vi "Multiclamp Capacitance Compensation.vi"(7 "#i":i32, 8 "error in (no error)":errorcluster, 9 "Timeout [ms]":u32, 10 "pnError":i32, 11 "hMCCmsg":i32) -> (0 "error out":errorcluster, 2 "pnError out":i32, 3 "Handler":i32)   [LabVIEW 2012, in "MultiClamp 700B Controls.lvlib"]
uses:
  MultiClamp 700B Controls.lvlib
  AxMultiClampMsg/AxMultiClampMsg.lvlib
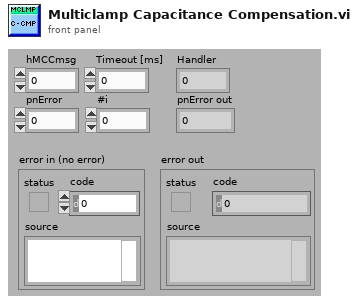
[diagram p1: front panel]
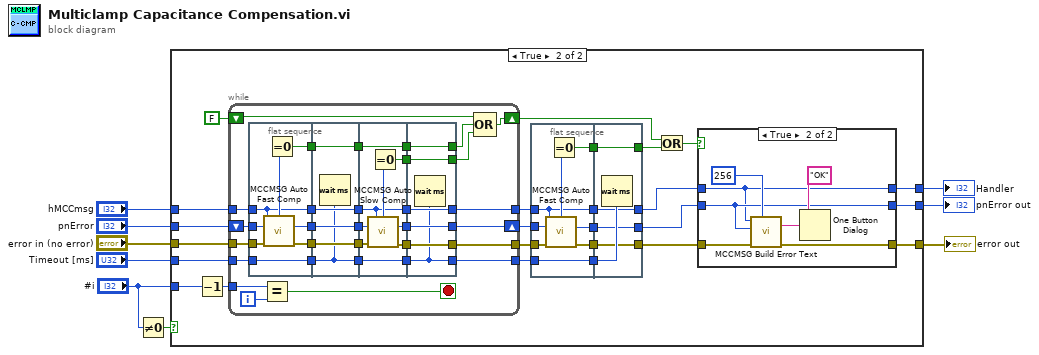
[diagram p0: block diagram]
diagram:
  n1 = Not Equal To 0?(x="#i") -> (x != 0?=w2:bool)
  n2 = case shown="True" w2 {
    tunnel: [w12 w32] -> w9
    tunnel: [w11 w31] -> w8
    tunnel: [w10 w30] -> w7
    tunnel: "error in (no error)" -> [w12 w29]
    tunnel: "pnError" -> [w10 w28]
    tunnel: "Timeout [ms]" -> [_ w27]
    tunnel: "#i" -> [_ w15]
    tunnel: "hMCCmsg" -> [w11 w13]
    frame False {
    }
    frame True {
      n3 = Decrement(x=w15) -> (x-1=w14:i32)
      n4 = while {
        tunnel: [w54] -> w25
        tunnel: [w52] -> w19
        tunnel: w29 -> [w63]
        tunnel: w13 -> [w62]
        tunnel: w27 -> [w60]
        tunnel: w14 -> [w59]
        shift-right: [w53] -> w23
        shift-left: w28 -> [w61]
        shift-right: [w56] -> w18
        shift-left: FALSE -> [w55]
        tunnel: [w51] -> w24
        i -> [w58]
        stop <- w57 stop-if-true
        n5 = flat-sequence {
          tunnel: [w89] -> w81
          tunnel: [w88] -> w80
          tunnel: w62 -> [w83]
          tunnel: w61 -> [w87]
          tunnel: w63 -> [w86]
          tunnel: [w84] -> w79
          tunnel: [w83] -> w78
          tunnel: w60 -> [w82]
          tunnel: [w82] -> w77
          tunnel: [w94] -> w76
          tunnel: w81 -> [w94]
          tunnel: w80 -> [w93]
          tunnel: [w93] -> w75
          tunnel: [w92] -> w74
          tunnel: w79 -> [w92]
          tunnel: [w91] -> w73
          tunnel: w78 -> [w91]
          tunnel: w77 -> [w90]
          tunnel: [w90] -> w72
          tunnel: w76 -> [w103]
          tunnel: [w102] -> w71
          tunnel: [w101] -> w70
          tunnel: w75 -> [w100]
          tunnel: [w98] -> w69
          tunnel: w74 -> [w98]
          tunnel: [w97] -> w68
          tunnel: w73 -> [w96]
          tunnel: [w96] -> w67
          tunnel: w72 -> [w95]
          tunnel: [w95] -> w66
          tunnel: w71 -> [w107]
          tunnel: w70 -> [w106]
          tunnel: w69 -> [w109]
          tunnel: w68 -> [w108]
          tunnel: w67 -> [w105]
          tunnel: w66 -> [w104]
          tunnel: [w109] -> w65
          tunnel: [w108] -> w64
          tunnel: [w107] -> w54
          tunnel: [w106] -> w53
          tunnel: [w105] -> w52
          tunnel: [w104] -> w51
          frame #0 {
            n6 = call "MCCMSG Auto Fast Comp.vi"("error in (no error)"=w86, "pnError"=w87, "hMCCmsg"=w83) -> ("error out"=w89:errorcluster, "pnError out"=w88:i32, "function return"=w85:i32)  [unwired: 6 in]
            n7 = Equal To 0?(x=w85) -> (x = 0?=w84:bool)
          }
          frame #1 {
            n8 = Wait (ms)(milliseconds to wait=w90) -> ()  [unwired: 1 out]
          }
          frame #2 {
            n9 = call "MCCMSG Auto Slow Comp.vi"("error in (no error)"=w103, "pnError"=w100, "hMCCmsg"=w96) -> ("error out"=w102:errorcluster, "pnError out"=w101:i32, "function return"=w99:i32)  [unwired: 6 in]
            n10 = Equal To 0?(x=w99) -> (x = 0?=w97:bool)
          }
          frame #3 {
            n11 = Wait (ms)(milliseconds to wait=w104) -> ()  [unwired: 1 out]
          }
        }
        n12 = Equal?(x=w59, y=w58) -> (x = y?=w57:bool)
        n13 = Compound Arithmetic op=OR(w55, w65, w64) -> (w56:bool)
      }
      n14 = flat-sequence {
        tunnel: [w45] -> w37
        tunnel: [w44] -> w36
        tunnel: w19 -> [w39]
        tunnel: w23 -> [w43]
        tunnel: w25 -> [w42]
        tunnel: [w40] -> w35
        tunnel: [w39] -> w34
        tunnel: w24 -> [w38]
        tunnel: [w38] -> w33
        tunnel: w37 -> [w48]
        tunnel: w36 -> [w47]
        tunnel: w35 -> [w50]
        tunnel: w34 -> [w46]
        tunnel: w33 -> [w49]
        tunnel: [w50] -> w17
        tunnel: [w48] -> w22
        tunnel: [w47] -> w21
        tunnel: [w46] -> w20
        frame #0 {
          n15 = call "MCCMSG Auto Fast Comp.vi"("error in (no error)"=w42, "pnError"=w43, "hMCCmsg"=w39) -> ("error out"=w45:errorcluster, "pnError out"=w44:i32, "function return"=w41:i32)  [unwired: 6 in]
          n16 = Equal To 0?(x=w41) -> (x = 0?=w40:bool)
        }
        frame #1 {
          n17 = Wait (ms)(milliseconds to wait=w49) -> ()  [unwired: 1 out]
        }
      }
      n18 = Or(x=w18, y=w17) -> (x .or. y?=w16:bool)
      n19 = case shown="True" w16 {
        tunnel: w21 -> [w112 w115]
        tunnel: w22 -> [w110 w119]
        tunnel: w20 -> [w111 w114]
        tunnel: [w112 w115] -> w30
        tunnel: [w111 w114] -> w31
        tunnel: [w110 w113] -> w32
        frame False {
        }
        frame True {
          n20 = call "MCCMSG Build Error Text.vi"("uMaxLen"=u32 256, "error in (no error)"=w119, "nErrorNum"=w115, "hMCCmsg"=w114) -> ("error out"=w113:errorcluster, "sTxtBuf out"=w118:string)  [unwired: 5 in, 1 out]
          n21 = One Button Dialog(message=w118, button name ("OK")="OK") -> ()  [unwired: 1 out]
        }
      }
    }
  }
  "error out" <- w9
  "Handler" <- w8
  "pnError out" <- w7
